vi "compile streams into async fifos.vi"(8 "error in":errorcluster, 11 "CD in":T1 format="%.0x") -> (0 "error out":errorcluster, 2 "compiled stream data":T3={"stream name"="", "Base URL"="https://api.gov.nominal.io/api/", "api key"="", "identifier selection"=enum."Asset Identifier and Dataset Name", "asset ID"="", "dataset name"="", "dataset ID"="", "associated channels"=[], "fallback avro path"=path "", "time source"=enum."to timestamp", "buffer size"=0}, 3 "fifo groups":T2(array[cluster]) {"VS Refs" format="%.0x"})   [LabVIEW 2026, in "Nominal Core Streaming System Explorer.lvlib"]
uses:
  Nominal Core Streaming System Explorer.lvlib
  Shared/compiled stream data.ctl
  Shared/stream configuration mode.ctl
  Shared/time convert type.ctl
  <vilib>/NI VeriStand/Custom Device API/Custom Device Item Ref.ctl
  <vilib>/NI VeriStand/Custom Device API/Custom Device API.lvlib
  Shared/Nominal Core Streaming Shared.lvlib
  <vilib>/Utility/SystemLogging/NI_SystemLogging.lvlib
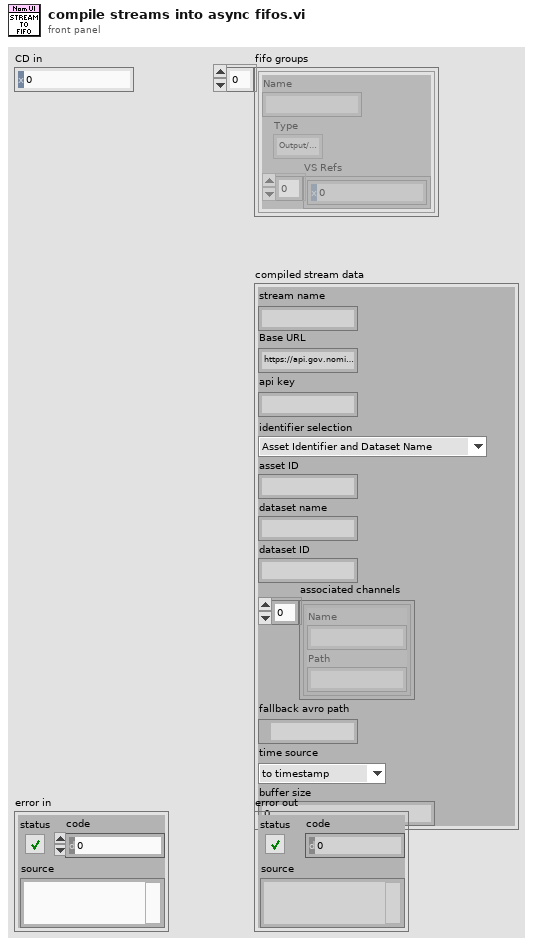
[diagram p1: front panel]
types:
  T1 = typedef "Custom Device API.lvlib/Custom Device Item Ref.ctl" = u64
  T2 = cluster{"Name":string, "Type":enum16{"Output/Write", "Input/Read", "Input/ReadWrite"}, "VS Refs":T1[]}[]
  T3 = typedef "Nominal Core Streaming Shared.lvlib/compiled stream data.ctl" = cluster{"stream name":string, "Base URL":string, "api key":string, "identifier selection":T4, "asset ID":string, "dataset name":string, "dataset ID":string, "associated channels":cluster{"Name":string, "Path":string}[], "fallback avro path":path, "time source":T5, "buffer size":u32}
  T4 = typedef "Nominal Core Streaming Shared.lvlib/stream configuration mode.ctl" = enum16{"Asset Identifier and Dataset Name", "Dataset Identifier"}
  T5 = typedef "Nominal Core Streaming Shared.lvlib/time convert type.ctl" = enum16{"to timestamp", "relative seconds"}
  T6 = enum16{"Output/Write", "Input/Read", "Input/ReadWrite"}
  T7 = cluster{"Name":string, "Type":enum16{"Output/Write", "Input/Read", "Input/ReadWrite"}, "VS Refs":T1[]}
  T8 = typedef "Custom Device API.lvlib/Custom Device Item Info.ctl" = cluster{"Name":string, "Is Channel":bool, "GUID":string, "Is Waveform":bool}
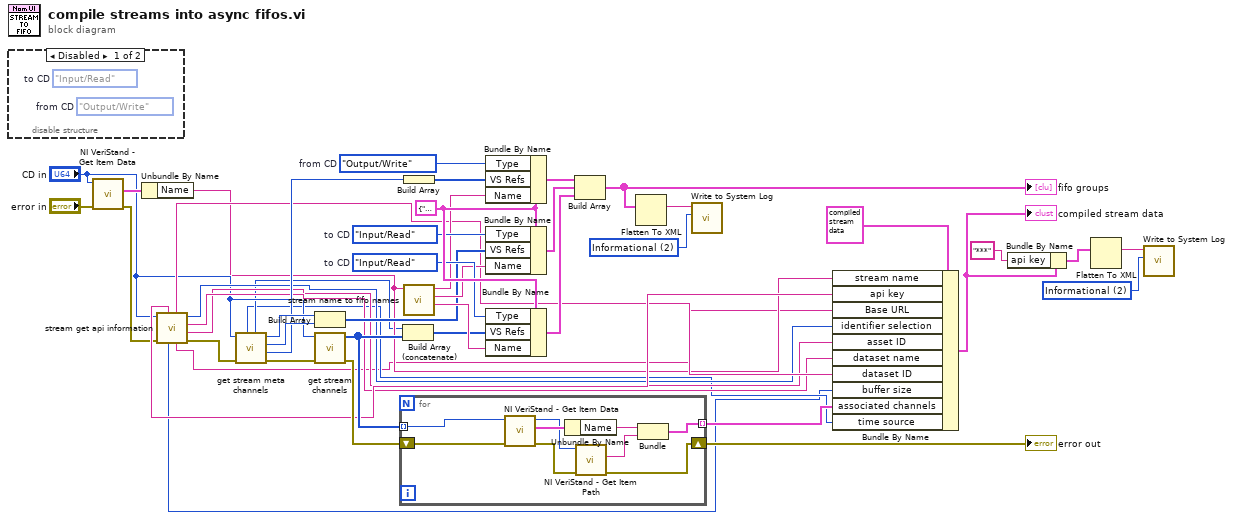
[diagram p0: block diagram]
diagram:
  w32 = T6."Input/Read"  # to CD
  w33 = T6."Input/Read"  # to CD
  w34 = T6."Output/Write"  # from CD
  w38 = T7 {"Name"="", "Type"=enum."Output/Write", "VS Refs"=[]} ("Group")
  w41 = 2 items=["Error", "Warning", "Informational"] ("severity")
  w43 = 2 items=["Error", "Warning", "Informational"] ("severity")
  n1 = disable-structure shown="Disabled" {
    frame Disabled {
      (unwired) T6."Input/Read"  # to CD
      (unwired) T6."Output/Write"  # from CD
    }
    frame Enabled {
    }
  }
  n2 = call <vilib>:"NI VeriStand - Get Item Data.vi"("error in (no error)"="error in", "Item Ref in"="CD in") -> ("error out"=w14:errorcluster, "Item Info"=w13:T8)  [unwired: 6 in, 2 out]
  n3 = Unbundle By Name(w13) -> ("Name"=w5:string)
  n4 = call "stream get api information.vi"("error in"=w14, "CD in"="CD in") -> ("error out"=w8:errorcluster, "asset ID"=w9:string, "dataset name"=w10:string, "ID selection"=w11:T4, "nominal base url"=w2:string, "dataset ID"=w12:string, "Channel buffer size"=w1:u32, "API key"=w15:string)  [unwired: 2 in]
  n5 = call "get stream meta channels.vi"("error in"=w8, "stream ref in"="CD in") -> ("error out"=w39:errorcluster, "status (out) channel"=w24:T1, "decimation (in) channel"=w25:T1, "enable (in) channel"=w26:T1, "time (in) channel"=w4:T1, "time source"=w3:T5)  [unwired: 4 in]
  n6 = Build Array(w26, w25) -> (w28:T1[])
  n7 = call "get stream channels.vi"("error in (no error)"=w39, "Item Ref in"="CD in") -> ("error out"=w23:errorcluster, "Dependent Node Refs"=w22:T1[])  [unwired: 8 in]
  n8 = for {
    shift-right: [w51] -> w45
    shift-left: w23 -> [w54]
    tunnel: w22 -> [w52] mode=indexing
    tunnel: [w46] -> w6 mode=indexing
    n9 = call <vilib>:"NI VeriStand - Get Item Data.vi"("error in (no error)"=w54, "Item Ref in"=w52) -> ("error out"=w53:errorcluster, "Item Info"=w50:T8, "Item Ref out"=w49:T1)  [unwired: 6 in, 1 out]
    n10 = Unbundle By Name(w50) -> ("Name"=w47:string)
    n11 = call <vilib>:"NI VeriStand - Get Item Path.vi"("error in (no error)"=w53, "Item Ref in"=w49) -> ("error out"=w51:errorcluster, "Path"=w48:string)  [unwired: 6 in, 2 out]
    n12 = Bundle("Name"=w47, "Path"=w48) -> (w46:cluster{"Name":string, "Path":string})  [unwired: 1 in]
  }
  "error out" <- w45
  n13 = Build Array (concatenate)(w4, w22) -> (w21:T1[])
  n14 = Build Array(w24) -> (w27:T1[])
  n15 = call "stream name to fifo names.vi"("Name"=w5) -> ("data to CD"=w29:string, "meta to CD"=w30:string, "meta from CD"=w31:string)  [unwired: 8 in]
  n16 = Bundle By Name(cluster=w38, "Type"=w34, "VS Refs"=w27, "Name"=w31) -> (w35:T7)
  n17 = Bundle By Name(cluster=w38, "Type"=w33, "VS Refs"=w28, "Name"=w30) -> (w36:T7)
  n18 = Bundle By Name(cluster=w38, "Type"=w32, "VS Refs"=w21, "Name"=w29) -> (w37:T7)
  n19 = Build Array(w35, w36, w37) -> (w42:T2)
  "fifo groups" <- w42
  n20 = Flatten To XML(6:w42) -> (2:w44:string)
  n21 = call <vilib>:"Write to System Log.vi"("severity"=w43, "message"=w44) -> ()  [unwired: 9 in, 1 out]
  n22 = Bundle By Name(cluster=T3 {"stream name"="", "Base URL"="https://api.gov.nominal.io/api/", "api key"="", "identifier selection"=enum."Asset Identifier and Dataset Name", "asset ID"="", "dataset name"="", "dataset ID"="", "associated channels"=[], "fallback avro path"=path "", "time source"=enum."to timestamp", "buffer size"=0} ("Cluster"), "stream name"=w5, "api key"=w15, "Base URL"=w2, "identifier selection"=w11, "asset ID"=w9, "dataset name"=w10, "dataset ID"=w12, "buffer size"=w1, "associated channels"=w6, "time source"=w3) -> (w18:T3)
  "compiled stream data" <- w18
  n23 = Bundle By Name(cluster=w18, "api key"="***") -> (w17:T3)
  n24 = Flatten To XML(6:w17) -> (2:w40:string)
  n25 = call <vilib>:"Write to System Log.vi"("severity"=w41, "message"=w40) -> ()  [unwired: 9 in, 1 out]
